vi "DeviceInfo.vi"(8 "Error in":errorcluster, 11 "Device":refnum<k24>) -> (0 "Error out":errorcluster, 2 "DeviceInfo":T1, 3 "Device":refnum<k24>)   [LabVIEW 2016]
doc: "Delivers various device properties.\n\nDevice: Device whose properties should be read\nDeviceInfo: Cluster that contains information about the device"
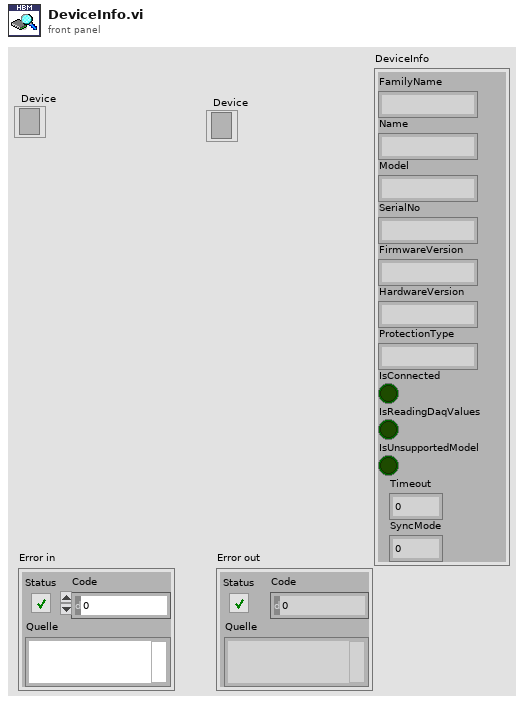
[diagram p1: front panel]
types:
  T1 = cluster{"FamilyName":string, "Name":string, "Model":string, "SerialNo":string, "FirmwareVersion":string, "HardwareVersion":string, "ProtectionType":string, "IsConnected":bool, "IsReadingDaqValues":bool, "IsUnsupportedModel":bool, "Timeout":i32, "SyncMode":i32}
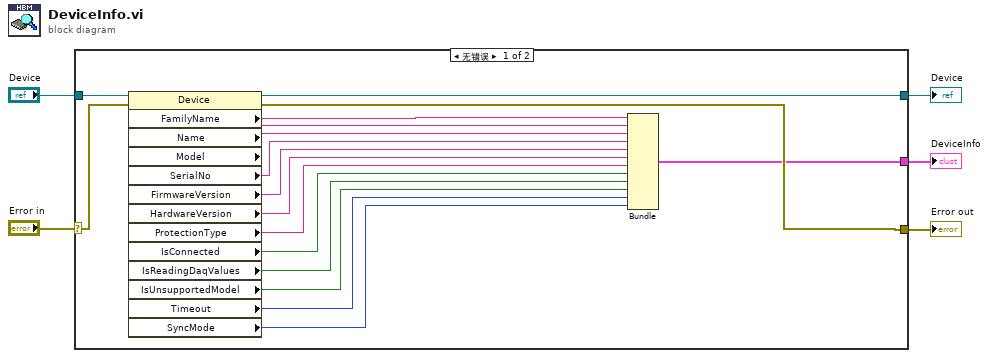
[diagram p0: block diagram]
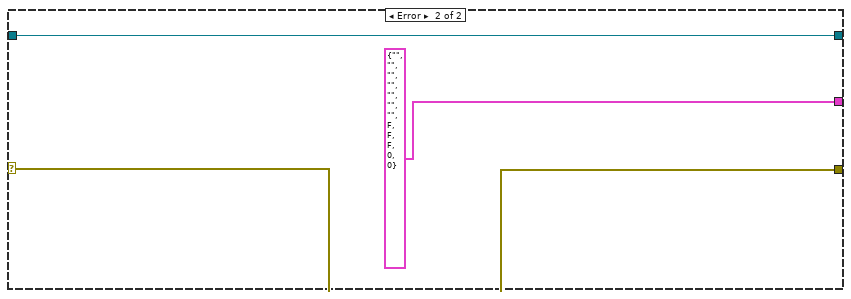
[diagram p2: hidden frame]
diagram:
  n1 = case shown="无错误" "Error in" {
    selector: "Error in" -> [w19 w24]
    tunnel: [w7 w24] -> w5
    tunnel: "Device" -> [w8 w23]
    tunnel: [w8 w23] -> w2
    tunnel: [w6 T1 {"FamilyName"="", "Name"="", "Model"="", "SerialNo"="", "FirmwareVersion"="", "HardwareVersion"="", "ProtectionType"="", "IsConnected"=FALSE, "IsReadingDaqValues"=FALSE, "IsUnsupportedModel"=FALSE, "Timeout"=0, "SyncMode"=0}] -> w1
    frame No Error {
      n2 = property on="Eigenschaftsknoten" class="Device"(reference=w8, error in=w19) -> (error out=w7:errorcluster, "FamilyName"=w21:string, "Name"=w20:string, "Model"=w18:string, "SerialNo"=w17:string, "FirmwareVersion"=w16:string, "HardwareVersion"=w15:string, "ProtectionType"=w14:string, "IsConnected"=w13:bool, "IsReadingDaqValues"=w12:bool, "IsUnsupportedModel"=w11:bool, "Timeout"=w10:i32, "SyncMode"=w9:i32)  [unwired: 1 out]
      n3 = Bundle("FamilyName"=w21, "Name"=w20, "Model"=w18, "SerialNo"=w17, "FirmwareVersion"=w16, "HardwareVersion"=w15, "ProtectionType"=w14, "IsConnected"=w13, "IsReadingDaqValues"=w12, "IsUnsupportedModel"=w11, "Timeout"=w10, "SyncMode"=w9) -> (w6:T1)  [unwired: 1 in]
    }
    frame Error {
    }
  }
  "Error out" <- w5
  "Device" <- w2
  "DeviceInfo" <- w1
